vi "Result.vi"(8 "error in (no error)":errorcluster, 10 "Result":T1={"Name"="", "Message"="", "Description"="", "Status"=enum."Passed", "Result Type"=enum."Test Suite", "Execution Time"=0.0}, 11 "Execution API In":refnum<class "Execution API.lvclass">) -> (0 "error out":errorcluster)   [LabVIEW 2020, in "Execution API.lvclass"]
uses:
  Execution API.lvclass
  Core/Result/Result.ctl
  Core/Result/Status.ctl
  Core/Result/Type.ctl
  Execution API.lvclass/Execution API.ctl
  Framework/Plugin/Plugin.lvclass
  Core/Result/Result.lvlib
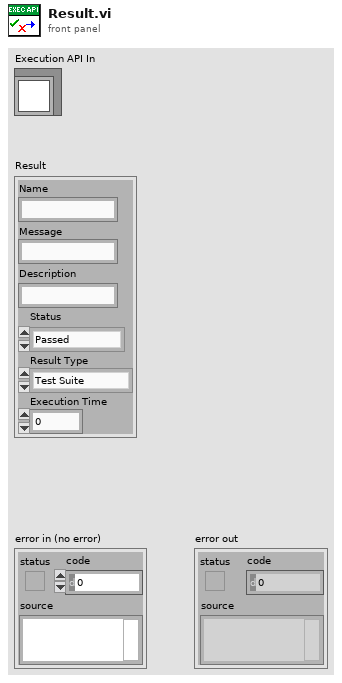
[diagram p1: front panel]
types:
  T1 = typedef "Result.lvlib/Result.ctl" = cluster{"Name":string, "Message":string, "Description":string, "Status":T2, "Result Type":T3, "Execution Time":dbl}
  T2 = typedef "Result.lvlib/Status.ctl" = enum16{"", "Passed", "Failed", "Error", "Skipped", "Setup Error", "Broken", "Teardown Error"}
  T3 = typedef "Result.lvlib/Type.ctl" = enum16{"Test Case", "Test Suite", "Test Run", "Pass", "Fail", "Skip", "Pass if", "Fail if", "Pass if Error", "Fail if Error", "Pass if Equal", "Fail if Equal"}
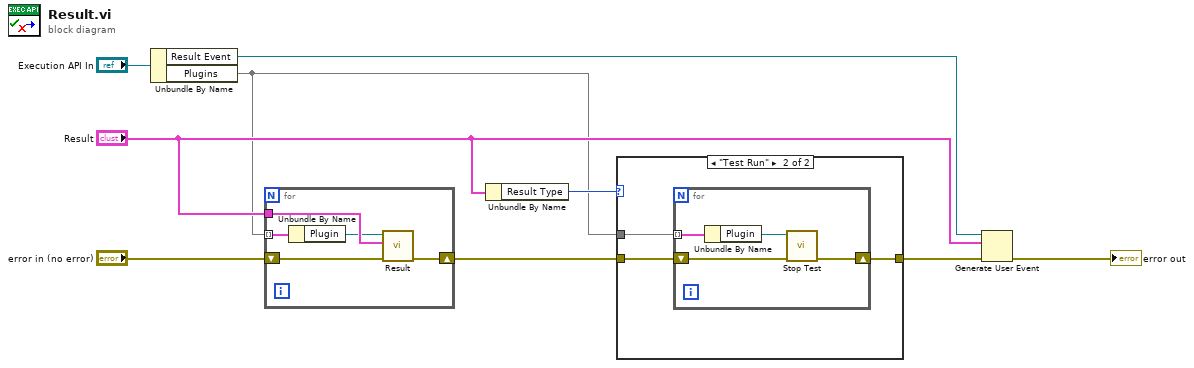
[diagram p0: block diagram]
diagram:
  n1 = Unbundle By Name("Execution API In") -> ("Result Event"=w8:refnum<user-event>, "Plugins"=w1:map{string, refnum<class "Plugin.lvclass">})
  n2 = for {
    tunnel: "Result" -> [w12]
    tunnel: w1 -> [w11] mode=indexing
    shift-right: [w13] -> w3
    shift-left: "error in (no error)" -> [w14]
    n3 = Unbundle By Name(w11) -> ("Plugin"=w10:refnum<class "Plugin.lvclass">)
    n4 = call-dynamic "Result.vi"("error in (no error)"=w14, "Result"=w12, "Plugin In"=w10) -> ("error out"=w13:errorcluster)  [unwired: 8 in]
  }
  n5 = Unbundle By Name("Result") -> ("Result Type"=w5:T3)
  n6 = case shown="\"Test Run\"" w5 {
    tunnel: w3 -> [w15 w18]
    tunnel: [w15 w17] -> w6
    tunnel: w1 -> [_ w16]
    frame Default {
    }
    frame "Test Run" {
      n7 = for {
        shift-right: [w21] -> w17
        shift-left: w18 -> [w22]
        tunnel: w16 -> [w20] mode=indexing
        n8 = Unbundle By Name(w20) -> ("Plugin"=w19:refnum<class "Plugin.lvclass">)
        n9 = call-dynamic "Stop Test.vi"("error in (no error)"=w22, "Plugin in"=w19) -> ("error out"=w21:errorcluster)  [unwired: 8 in, 1 out]
      }
    }
  }
  n10 = Generate User Event(user event=w8, event data cluster="Result", error in=w6) -> (error out=→"error out":errorcluster)  [unwired: 1 in, 1 out]
